vi "Calibration.vi"(8 "error in (no error)":errorcluster, 11 "Connection Data In":T2={"MX370x refnum"=refnum, "IP"="192.168.99.99", "Connection ID "=refnum, "MXCommon refnum"=refnum}) -> (0 "error out":errorcluster={"status"=TRUE, "code"=1172, "source"="Constructor Node Error creating instance of Uri in assembly System.Uri, System, Version=4.0.0.0, Culture=neutral, PublicKeyToken=b77a5c561934e089, (System.UriFormatException: Invalid URI: The hostname could not be parsed.) <append><b>System.UriFormatException</b> in MSX-E3701_dll.lvlib:Connection Open.vi->MSX-E3701_dll.lvlib:Calibration.vi"}, 3 "Connection Data Out":T2)   [LabVIEW 2014, in "MSX-E3701_dll.lvlib"]
doc: "Paanel Frontal que permite la calibracion de transductores."
uses:
  MSX-E3701_dll.lvlib
  Typedef/Connection Data.ctl
  E:/Repositorio Magnis/INF002/v0/Modules/HAL/Drivers/Sync/ADDI-DATA MSX-E3701/API/MX370x.dll
  MX370x.dll
  E:/Repositorio Magnis/INF002/v0/Modules/HAL/Drivers/Sync/ADDI-DATA MSX-E3701/API/MXCommon.dll
  MXCommon.dll
  Typedef/Calibration Data.ctl
  Typedef/Calibration Enum.ctl
panel:
  in  "Transducer Selection":u64
  in  "Desired Position":dbl format="%#_g[mm]"
  in  "Stop":bool
  out "Progress Bar":u64(slide) scale=0.0..5.0
  out "Measured value":dbl format="%#_g[mm]"
  out "Indicator":string="Leyendo los transductores de la base de datos."
  in  "Next":bool
  in  "Start":bool
  out "Cluster Calibration":T1
  # "TRANSDUCER CALIBRATION"
  # "Progress Bar"
  # "Information"
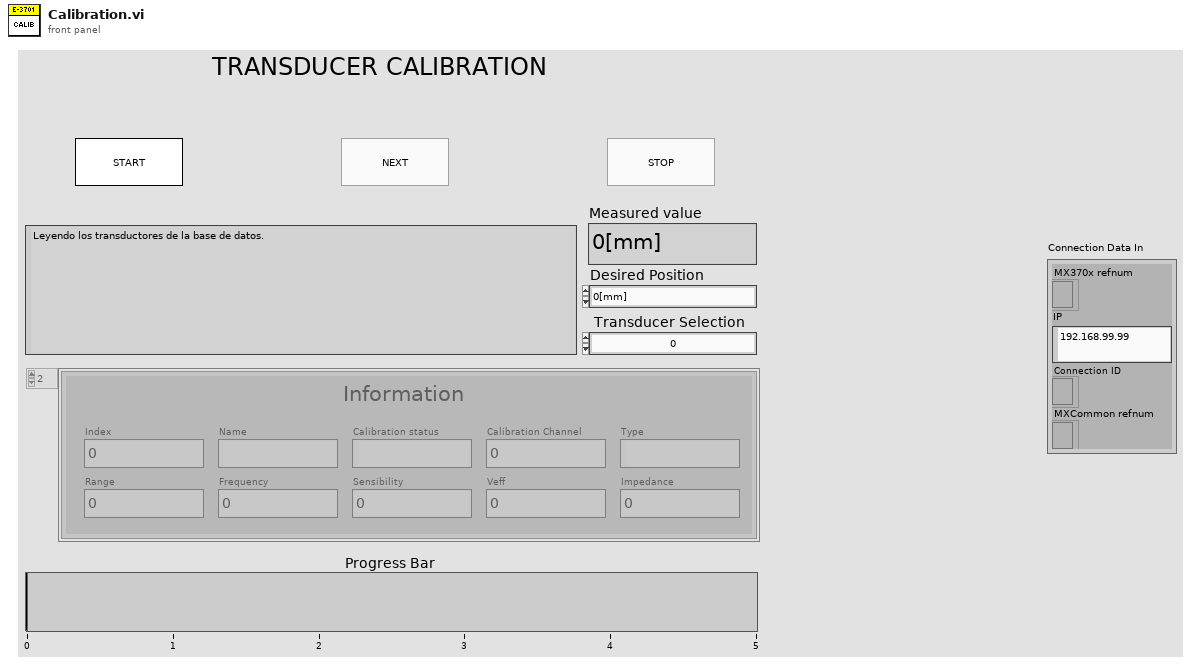
[diagram p1: front panel]
types:
  T1 = typedef "MSX-E3701_dll.lvlib/Calibration Data.ctl" = cluster{"Calibration status":string, "Name":string, "Index":u64, "Range":dbl, "Sensibility":dbl, "Veff":dbl, "Frequency":u64, "Impedance":u64, "Type":string, "Calibration Channel":u64}[]
  T2 = typedef "MSX-E3701_dll.lvlib/Connection Data.ctl" = cluster{"MX370x refnum":refnum<k24>, "IP":string, "Connection ID ":refnum<k5>, "MXCommon refnum":refnum<k24>}
  T3 = typedef "MSX-E3701_dll.lvlib/Calibration Enum.ctl" = enum16{"Init", "Idle Start", "Idle Next", "Open Web Service", "Read Transducers", "StartCalibration", "CalibrationGetCurrentStatus", "Save or Omit", "Close Web Service", "Idle Final"}
  T4 = enum8{"Enabled", "Disabled", "Disabled and Grayed Out"}
  T5 = cluster{"Calibration status":string, "Name":string, "Index":u64, "Range":dbl, "Sensibility":dbl, "Veff":dbl, "Frequency":u64, "Impedance":u64, "Type":string, "Calibration Channel":u64}
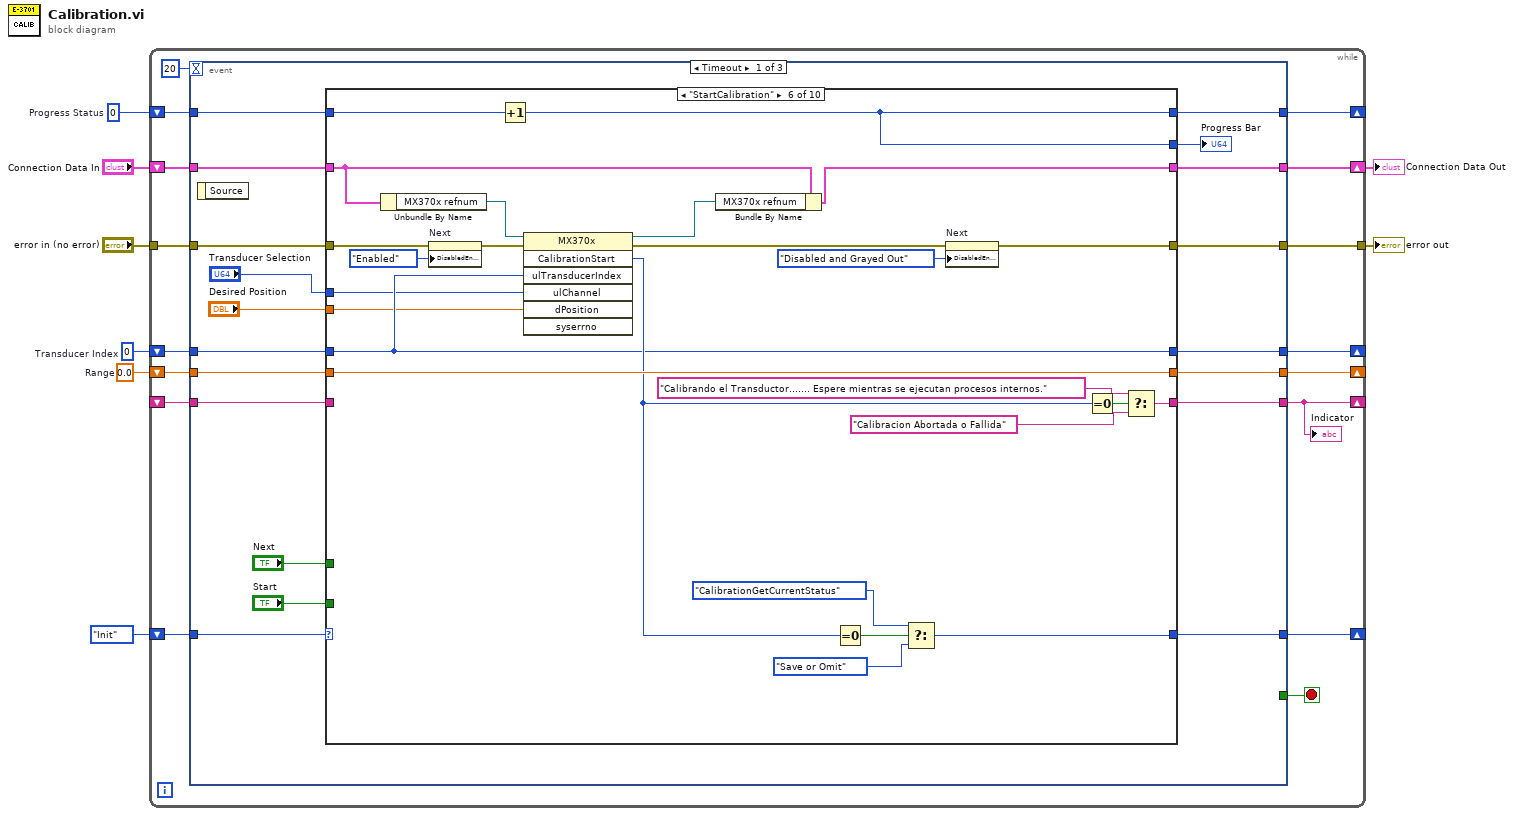
[diagram p0: block diagram]
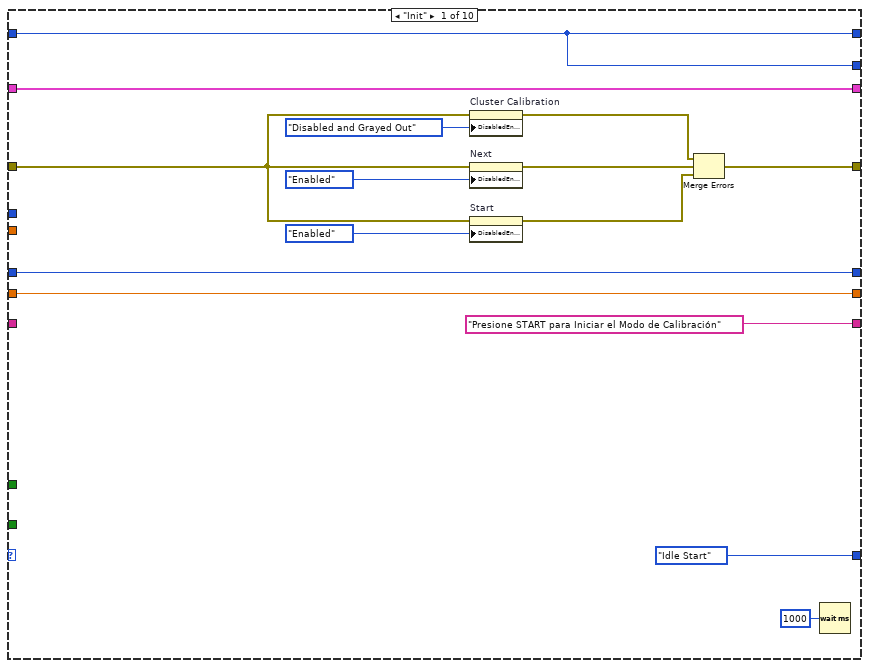
[diagram p2: hidden frame]
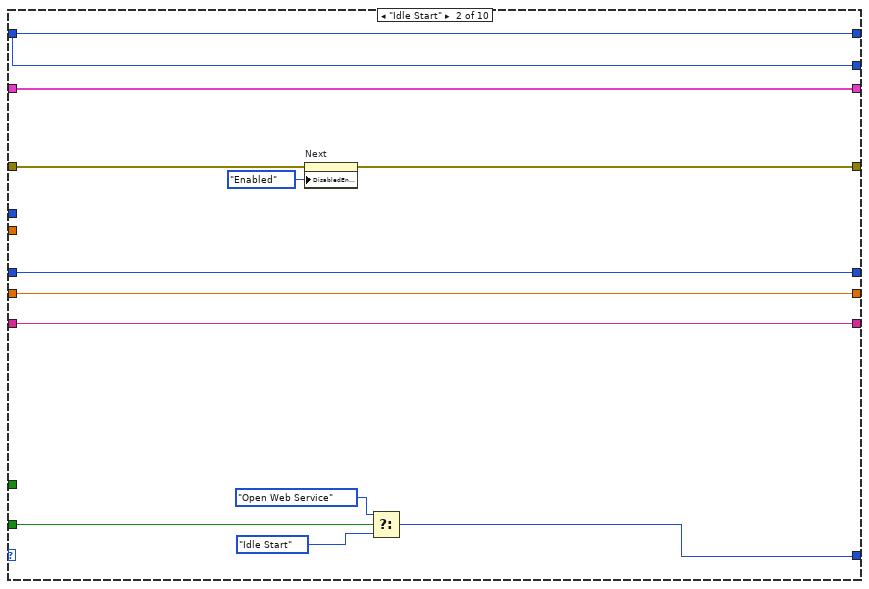
[diagram p3: hidden frame]
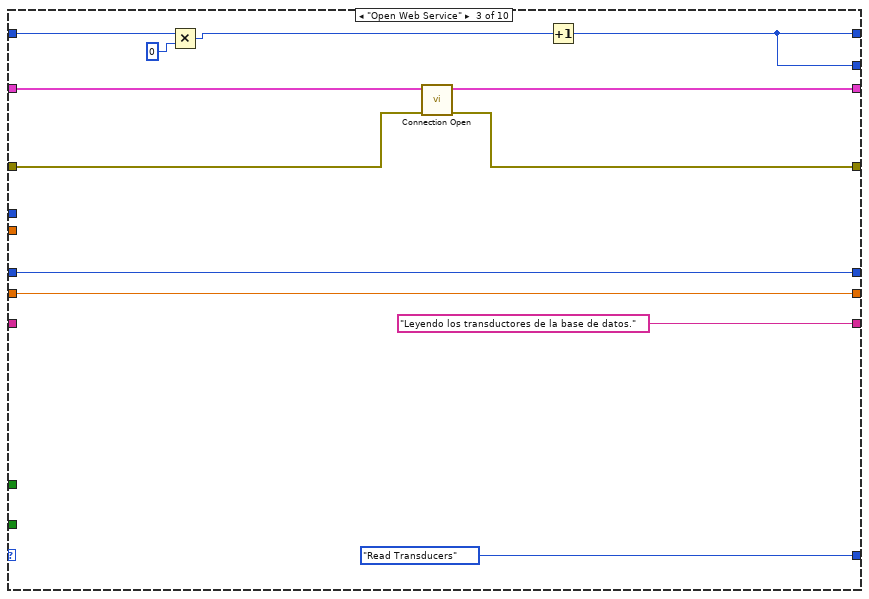
[diagram p4: hidden frame]
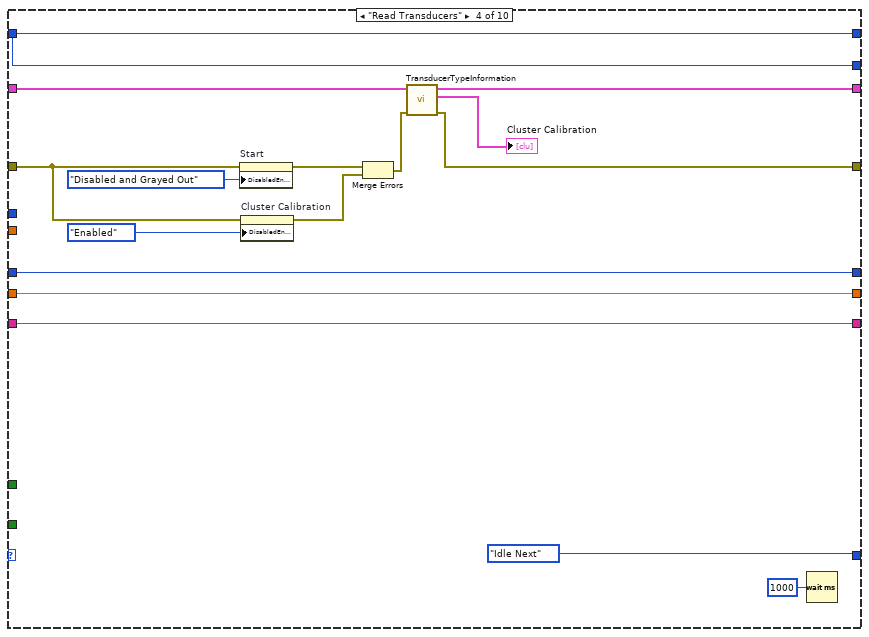
[diagram p5: hidden frame]
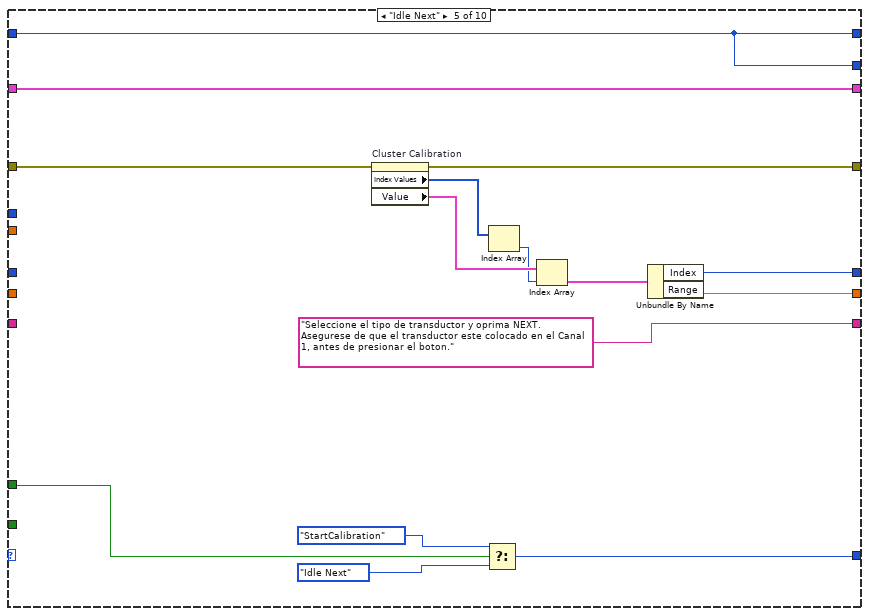
[diagram p6: hidden frame]
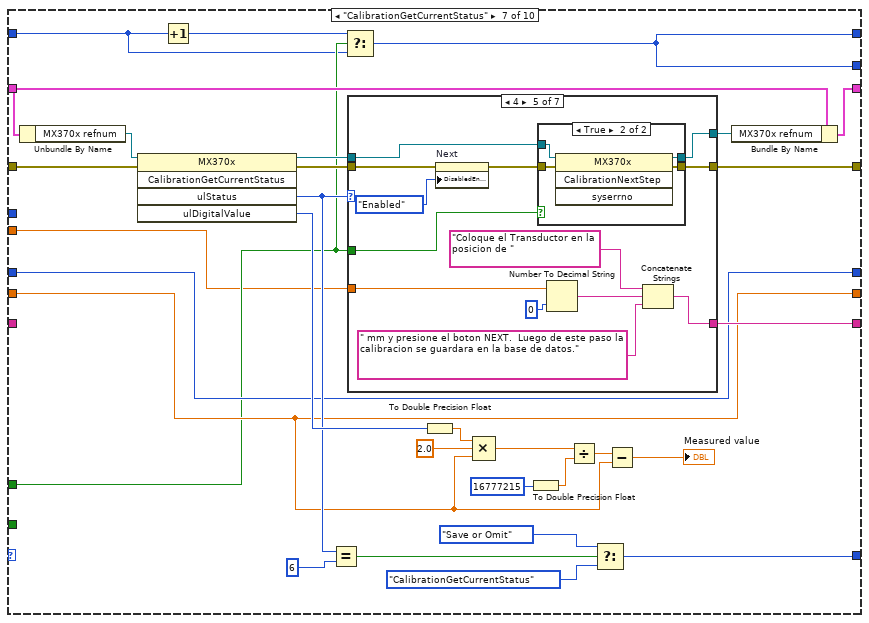
[diagram p7: hidden frame]
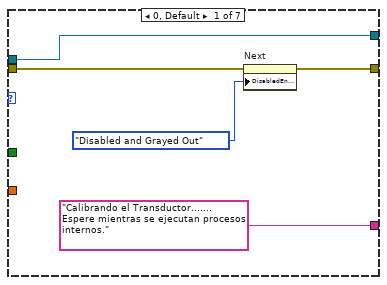
[diagram p8: hidden frame]
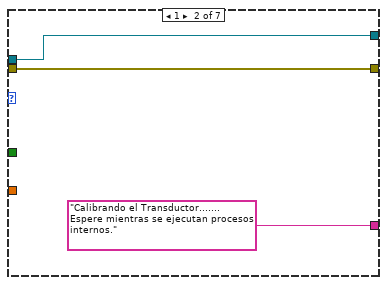
[diagram p9: hidden frame]
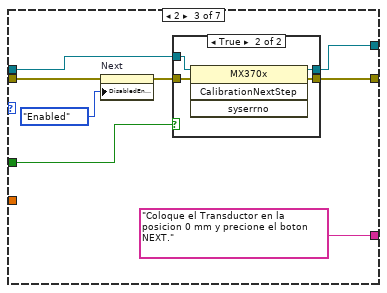
[diagram p10: hidden frame]
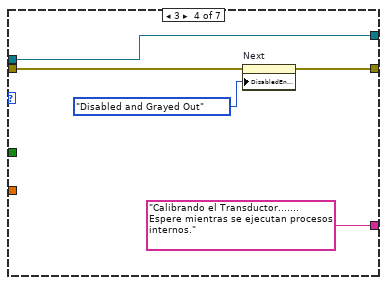
[diagram p12: hidden frame]
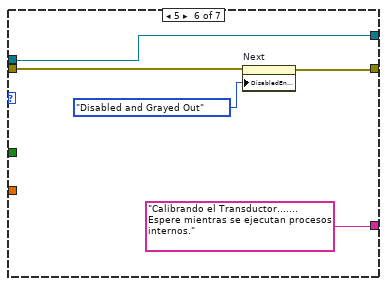
[diagram p14: hidden frame]
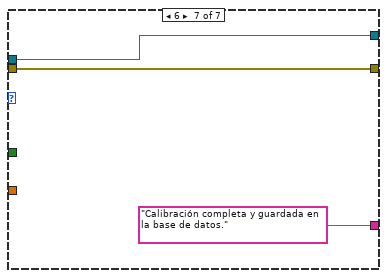
[diagram p15: hidden frame]
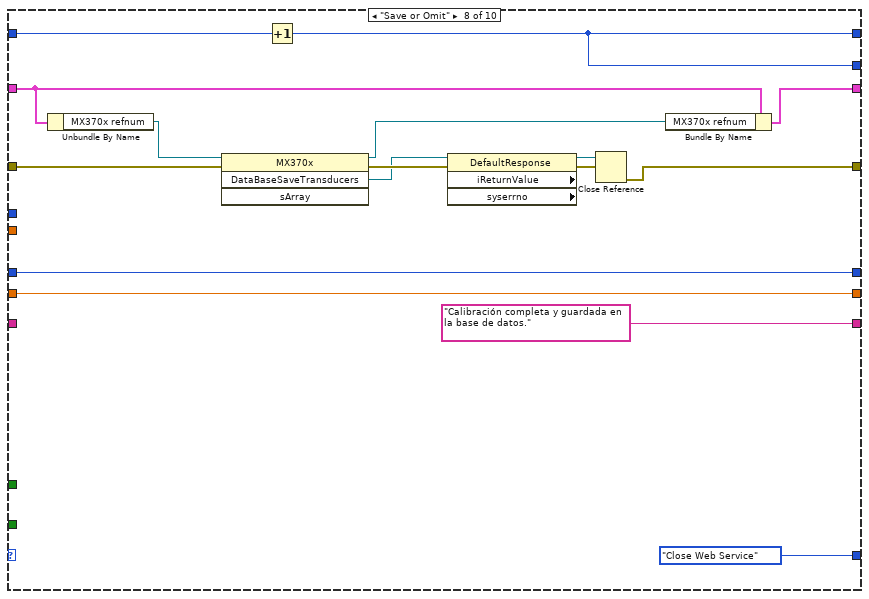
[diagram p16: hidden frame]
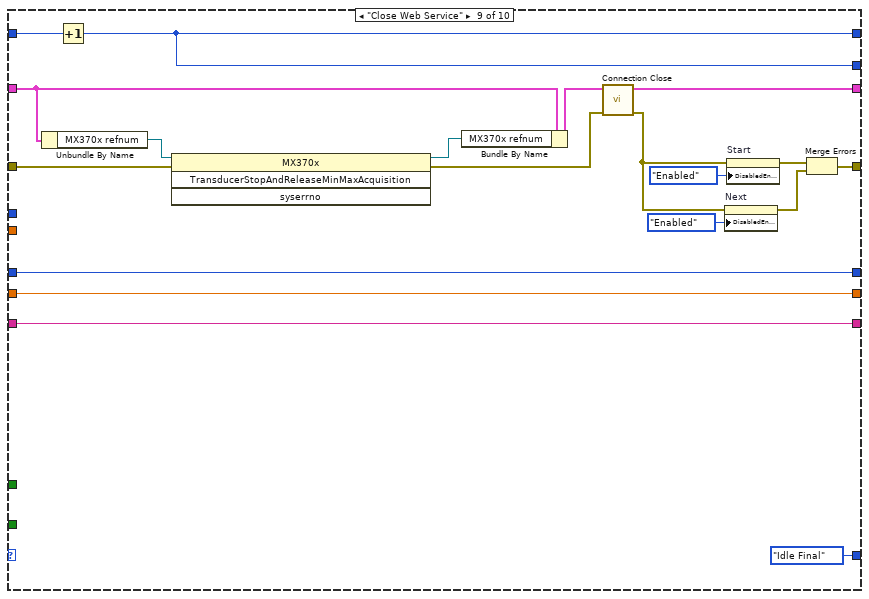
[diagram p17: hidden frame]
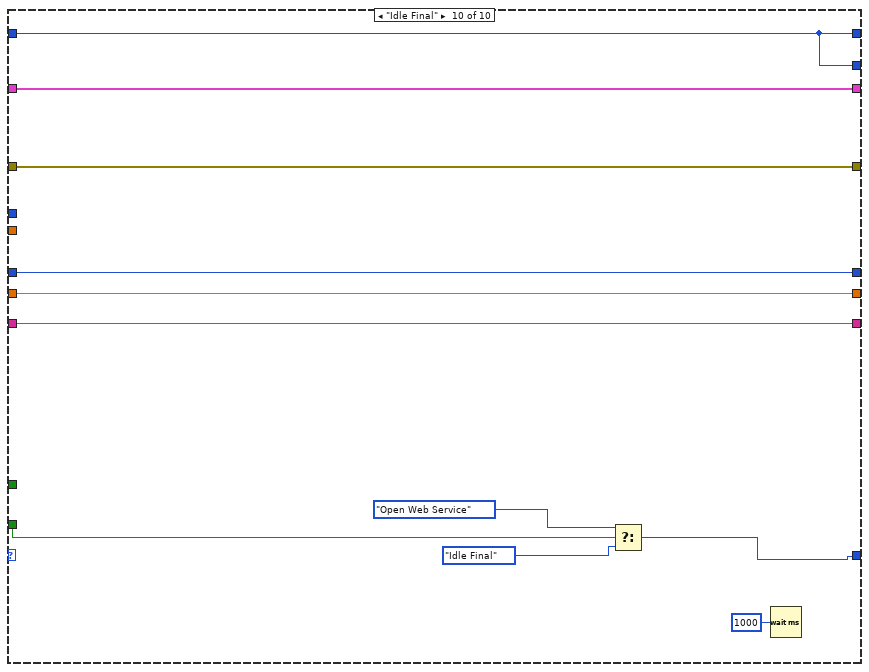
[diagram p18: hidden frame]
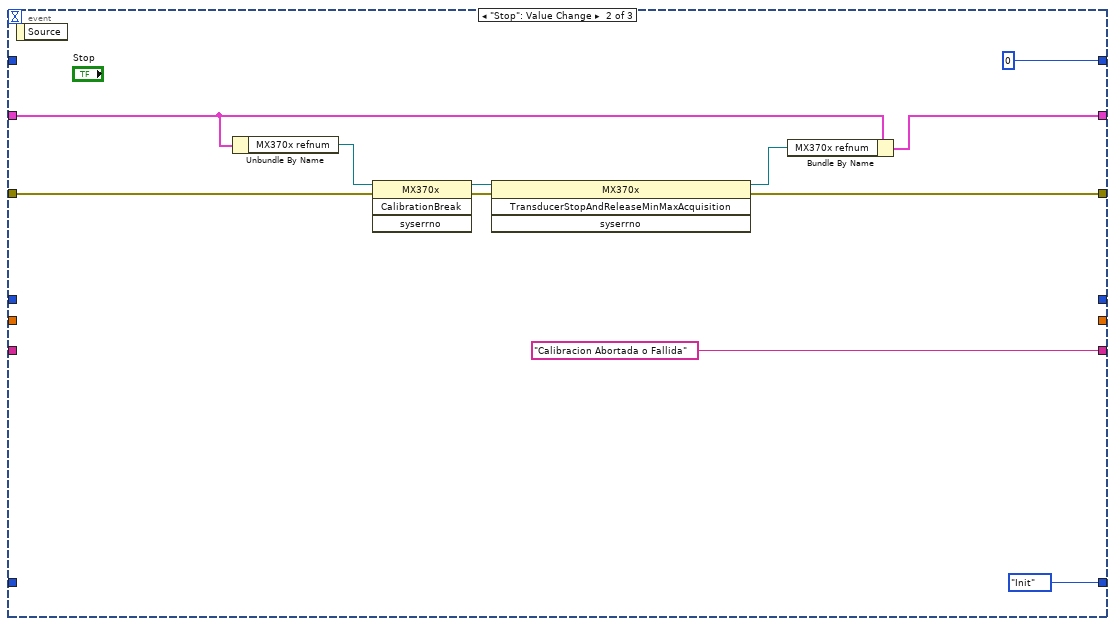
[diagram p19: hidden frame]
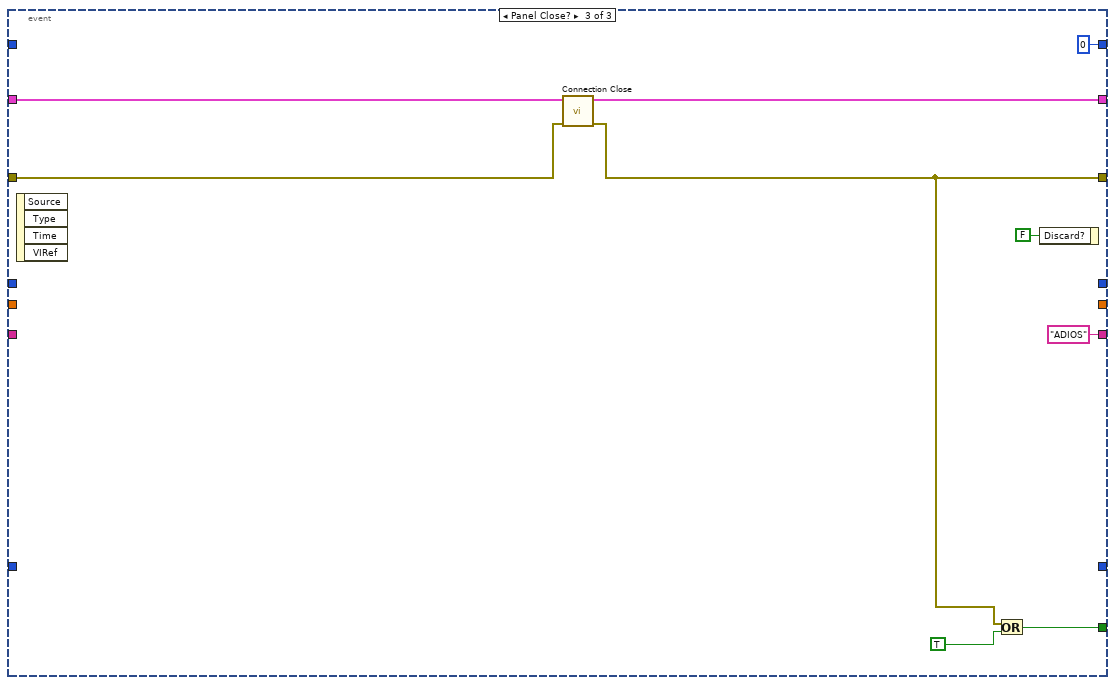
[diagram p20: hidden frame]
diagram:
  w1 = u64 0  # Progress Status
  w2 = 0.0  # Range
  w3 = u64 0  # Transducer Index
  n1 = while {
    tunnel: [w20] -> w6
    tunnel: "error in (no error)" -> [w22]
    shift-right: [w23] -> w7
    shift-left: "Connection Data In" -> [w24]
    shift-right: [w14] -> _
    shift-left: Calibration_Enum."Init" ("Enum") -> [w19]
    shift-right: [w18] -> _
    shift-left: w3 -> [w16]
    shift-right: [w17] -> _
    shift-left: w2 -> [w15]
    shift-right: [w12] -> _
    shift-left: w1 -> [w13]
    shift-right: [w10] -> _
    shift-left: _ -> [w9]
    stop <- w21 stop-if-true
    n2 = event shown="[0] Timeout" {
      selector: _ -> [_ _ _]
      dyn-events: _ -> [_ _ _]
      timeout: 20 -> [_ _ _]
      tunnel: w24 -> [w43 w278 w285]
      tunnel: [w42 w277 w284] -> w23
      tunnel: w22 -> [w41 w276 w283]
      tunnel: [_ _ w286] -> w21
      tunnel: [w40 w270 w282] -> w20
      tunnel: w19 -> [w38 _ _]
      tunnel: [w37 _ _] -> w18
      tunnel: [w36 _ _] -> w17
      tunnel: w16 -> [w35 _ _]
      tunnel: w15 -> [w34 _ _]
      tunnel: [w33 Calibration_Enum."Init" ("Enum") _] -> w14
      tunnel: w13 -> [w31 _ _]
      tunnel: [w30 u64 0 ("Progress Status") u64 0 ("Progress Status")] -> w12
      tunnel: [w28 "Calibracion Abortada o Fallida" ("Caption.Text") "ADIOS" ("Caption.Text")] -> w10
      tunnel: w9 -> [w27 _ _]
      event Timeout {
        n3 = event-data() -> ()  [unwired: 1 in, 1 out]
        n4 = case shown="\"StartCalibration\"" w38 {
          tunnel: w43 -> [w54 w70 w82 w98 w110 w137 w168 w236 w243 w268]
          tunnel: [w54 w70 w81 w97 w110 w135 w167 w235 w257 w268] -> w42
          tunnel: [w55 w61 w80 w96 w109 w117 w149 w234 w247 w267] -> w40
          tunnel: w41 -> [w50 w62 w79 w89 w100 w132 w166 w233 w245 w267]
          tunnel: [Calibration_Enum."Idle Start" ("Enum") w60 Calibration_Enum."Read Transducers" ("f") Calibration_Enum."Idle Next" ("Enum") w99 w116 w140 Calibration_Enum."Close Web Service" ("Enum") Calibration_Enum."Idle Final" ("Enum") w261] -> w33
          tunnel: "Start" -> [_ w68 _ _ _ _ _ _ _ w263]
          tunnel: [w48 w66 w78 w88 w102 w122 w145 w227 w255 w266] -> w37
          tunnel: [w47 w65 w77 w87 w107 w131 w146 w231 w254 w265] -> w36
          tunnel: w35 -> [w48 w66 w78 w88 _ w122 w145 w227 w255 w266]
          tunnel: w34 -> [w47 w65 w77 w87 _ w131 w146 w231 w254 w265]
          tunnel: ["Presione START para Iniciar el Modo de Calibración" ("Indicator") w59 "Leyendo los transductores de la base de datos." ("Indicator") w83 "Seleccione el tipo de transductor y oprima NEXT. Asegurese de que el transductor este colocado en el Canal 1, antes de presionar el boton." ("Caption.Text") w124 w147 "Calibración completa y guardada en la base de datos." ("Caption.Text") w239 w259] -> w28
          tunnel: "Next" -> [_ _ _ _ w103 _ w143 _ _ _]
          tunnel: [w46 w64 w75 w85 w101 w120 w144 w228 w240 w260] -> w30
          tunnel: w31 -> [w46 w64 w73 w85 w101 w121 w141 w229 w252 w260]
          tunnel: [w46 w64 w75 w85 w101 w120 w144 w228 w240 w260] -> w29
          tunnel: w27 -> [_ w59 _ w83 _ _ _ _ w239 w259]
          tunnel: "Desired Position" -> [_ _ _ _ _ w115 w139 _ _ _]
          tunnel: "Transducer Selection" -> [_ _ _ _ _ w114 _ _ _ _]
          frame "Init" {
            n5 = property on="Cluster Calibration" class="Arr (strict)"(error in=w50, "DisabledEnum"=T4."Disabled and Grayed Out" ("Disabled")) -> (error out=w56:errorcluster)  [unwired: 1 in, 1 out]
            n6 = property on="Next" class="Bool"(error in=w50, "DisabledEnum"=T4."Enabled" ("Disabled")) -> (error out=w52:errorcluster)  [unwired: 1 in, 1 out]
            n7 = property on="Start" class="Bool"(error in=w50, "DisabledEnum"=T4."Enabled" ("Disabled")) -> (error out=w51:errorcluster)  [unwired: 1 in, 1 out]
            n8 = Merge Errors(w56, w52, w51) -> (w55:errorcluster)
            n9 = Wait (ms)(milliseconds to wait=u32 1000) -> ()  [unwired: 1 out]
          }
          frame "Idle Start" {
            n10 = property on="Next" class="Bool"(error in=w62, "DisabledEnum"=T4."Enabled" ("Disabled")) -> (error out=w61:errorcluster)  [unwired: 1 in, 1 out]
            n11 = Select(t=Calibration_Enum."Open Web Service" ("Enum"), s=w68, f=Calibration_Enum."Idle Start") -> (s? t:f=w60:T3)
          }
          frame "Open Web Service" {
            n12 = Multiply(x=w73, y=u64 0) -> (x*y=w74:u64)
            n13 = call "Connection Open.vi"("Error In"=w79, "Connection Data In"=w82) -> ("Error Out"=w80:errorcluster, "Connection Data Out"=w81:T2)  [unwired: 8 in]
            n14 = Increment(x=w74) -> (x+1=w75:u64)
          }
          frame "Read Transducers" {
            n15 = property on="Start" class="Bool"(error in=w89, "DisabledEnum"=T4."Disabled and Grayed Out" ("Disabled")) -> (error out=w92:errorcluster)  [unwired: 1 in, 1 out]
            n16 = property on="Cluster Calibration" class="Arr (strict)"(error in=w89, "DisabledEnum"=T4."Enabled" ("Disabled")) -> (error out=w91:errorcluster)  [unwired: 1 in, 1 out]
            n17 = Merge Errors(w92, w91) -> (w90:errorcluster)
            n18 = call "TransducerTypeInformation.vi"("error in (no error)"=w90, "Connection Data In"=w98) -> ("error out"=w96:errorcluster, "Cluster Calibration"=→"Cluster Calibration":T1, "Connection Data Out"=w97:T2)  [unwired: 7 in]
            n19 = Wait (ms)(milliseconds to wait=u32 1000) -> ()  [unwired: 1 out]
          }
          frame "Idle Next" {
            n20 = property on="Cluster Calibration" class="Arr (strict)"(error in=w100) -> (error out=w109:errorcluster, "Index Values"=w113:u32[], "Value"=w112:T1)  [unwired: 1 in, 1 out]
            n21 = Select(t=Calibration_Enum."StartCalibration" ("Enum"), s=w103, f=Calibration_Enum."Idle Next") -> (s? t:f=w99:T3)
            n22 = Index Array(array=w113) -> (element=w108:u32)  [unwired: 1 in]
            n23 = Index Array(array=w112, index=w108) -> (element=w111:T5)
            n24 = Unbundle By Name(w111) -> ("Index"=w102:u64, "Range"=w107:dbl)
          }
          frame "StartCalibration" {
            n25 = Unbundle By Name(w137) -> ("MX370x refnum"=w138:refnum<k24>)
            n26 = property on="Next" class="Bool"(error in=w132, "DisabledEnum"=T4."Enabled" ("Disabled")) -> (error out=w133:errorcluster)  [unwired: 1 in, 1 out]
            n27 = Increment(x=w121) -> (x+1=w120:u64)
            n28 = invoke class="MX370x" method="CalibrationStart"(reference=w138, error in=w133, "ulTransducerIndex"=w122, "ulChannel"=w114, "dPosition"=w115) -> (reference out=w136:refnum<k24>, error out=w118:errorcluster, "CalibrationStart"=w126:i32)  [unwired: 2 in, 4 out]
            n29 = Bundle By Name(cluster=w137, "MX370x refnum"=w136) -> (w135:T2)
            n30 = Equal To 0?(x=w126) -> (x = 0?=w130:bool)
            n31 = Select(t=Calibration_Enum."CalibrationGetCurrentStatus" ("Enum"), s=w130, f=Calibration_Enum."Save or Omit" ("Enum")) -> (s? t:f=w116:T3)
            n32 = property on="Next" class="Bool"(error in=w118, "DisabledEnum"=T4."Disabled and Grayed Out" ("Disabled")) -> (error out=w117:errorcluster)  [unwired: 1 in, 1 out]
            n33 = Equal To 0?(x=w126) -> (x = 0?=w127:bool)
            n34 = Select(t="Calibrando el Transductor....... Espere mientras se ejecutan procesos internos." ("Caption.Text"), s=w127, f="Calibracion Abortada o Fallida") -> (s? t:f=w124:string)
          }
          frame "CalibrationGetCurrentStatus" {
            n35 = Unbundle By Name(w168) -> ("MX370x refnum"=w165:refnum<k24>)
            n36 = invoke class="MX370x" method="CalibrationGetCurrentStatus"(reference=w165, error in=w166) -> (reference out=w150:refnum<k24>, error out=w151:errorcluster, "ulStatus"=w156:u64, "ulDigitalValue"=w160:u64)  [unwired: 3 in, 1 out]
            n37 = Increment(x=w141) -> (x+1=w142:u64)
            n38 = Equal?(x=w156, y=u64 6) -> (x = y?=w154:bool)
            n39 = Select(t=w142, s=w143, f=w141) -> (s? t:f=w144:u64)
            n40 = case shown="4" w156 {
              tunnel: w151 -> [w172 w176 w179 w194 w204 w218 w220]
              tunnel: w150 -> [w170 w175 w180 w191 w205 w216 w222]
              tunnel: [w171 w176 w184 w193 w203 w217 w220] -> w149
              tunnel: [w170 w175 w183 w191 w197 w216 w222] -> w148
              tunnel: ["Calibrando el Transductor....... Espere mientras se ejecutan procesos internos." ("Caption.Text") "Calibrando el Transductor....... Espere mientras se ejecutan procesos internos." ("Caption.Text") "Coloque el Transductor en la posicion 0 mm y precione el boton NEXT." ("Caption.Text") "Calibrando el Transductor....... Espere mientras se ejecutan procesos internos." ("Caption.Text") w198 "Calibrando el Transductor....... Espere mientras se ejecutan procesos internos." ("Caption.Text") "Calibración completa y guardada en la base de datos." ("Caption.Text")] -> w147
              tunnel: w143 -> [_ _ w177 _ w206 _ _]
              tunnel: w139 -> [_ _ _ _ w196 _ _]
              frame 0, Default {
                n41 = property on="Next" class="Bool"(error in=w172, "DisabledEnum"=T4."Disabled and Grayed Out" ("Disabled")) -> (error out=w171:errorcluster)  [unwired: 1 in, 1 out]
              }
              frame 1 {
              }
              frame 2 {
                n42 = property on="Next" class="Bool"(error in=w179, "DisabledEnum"=T4."Enabled" ("Disabled")) -> (error out=w181:errorcluster)  [unwired: 1 in, 1 out]
                n43 = case shown="True" w177 {
                  tunnel: [w185 w190] -> w184
                  tunnel: [w186 w189] -> w183
                  tunnel: w181 -> [w185 w188]
                  tunnel: w180 -> [w186 w187]
                  frame False {
                  }
                  frame True {
                    n44 = invoke class="MX370x" method="CalibrationNextStep"(reference=w187, error in=w188) -> (reference out=w189:refnum<k24>, error out=w190:errorcluster)  [unwired: 2 in, 2 out]
                  }
                }
              }
              frame 3 {
                n45 = property on="Next" class="Bool"(error in=w194, "DisabledEnum"=T4."Disabled and Grayed Out" ("Disabled")) -> (error out=w193:errorcluster)  [unwired: 1 in, 1 out]
              }
              frame 4 {
                n46 = property on="Next" class="Bool"(error in=w204, "DisabledEnum"=T4."Enabled" ("Disabled")) -> (error out=w208:errorcluster)  [unwired: 1 in, 1 out]
                n47 = case shown="True" w206 {
                  tunnel: [w209 w214] -> w203
                  tunnel: [w210 w213] -> w197
                  tunnel: w208 -> [w209 w212]
                  tunnel: w205 -> [w210 w211]
                  frame False {
                  }
                  frame True {
                    n48 = invoke class="MX370x" method="CalibrationNextStep"(reference=w211, error in=w212) -> (reference out=w213:refnum<k24>, error out=w214:errorcluster)  [unwired: 2 in, 2 out]
                  }
                }
                n49 = Number To Decimal String(number=w196, width (-)=i16 0) -> (decimal integer string=w201:string)
                n50 = Concatenate Strings("Coloque el Transductor en la posicion de " ("Caption.Text"), w201, " mm y presione el boton NEXT.  Luego de este paso la calibracion se guardara en la base de datos.") -> (w198:string)
              }
              frame 5 {
                n51 = property on="Next" class="Bool"(error in=w218, "DisabledEnum"=T4."Disabled and Grayed Out" ("Disabled")) -> (error out=w217:errorcluster)  [unwired: 1 in, 1 out]
              }
              frame 6 {
              }
            }
            n52 = To Double Precision Float(number=w160) -> (double precision float=w159:dbl)
            n53 = Compound Arithmetic op=MULTIPLY(w159, 2.0 ("x"), w146) -> (w161:dbl)
            n54 = To Double Precision Float(number=u64 16777215 ("x")) -> (double precision float=w157:dbl)
            n55 = Divide(x=w161, y=w157) -> (x/y=w162:dbl)
            n56 = Select(t=Calibration_Enum."Save or Omit" ("Enum"), s=w154, f=Calibration_Enum."CalibrationGetCurrentStatus" ("Enum")) -> (s? t:f=w140:T3)
            n57 = Subtract(x=w162, y=w146) -> (x-y=→"Measured value":dbl)
            n58 = Bundle By Name(cluster=w168, "MX370x refnum"=w148) -> (w167:T2)
          }
          frame "Save or Omit" {
            n59 = Unbundle By Name(w236) -> ("MX370x refnum"=w238:refnum<k24>)
            n60 = invoke class="MX370x" method="DataBaseSaveTransducers"(reference=w238, error in=w233) -> (reference out=w237:refnum<k24>, error out=w224:errorcluster, "DataBaseSaveTransducers"=w223:refnum<k24>)  [unwired: 2 in, 1 out]
            n61 = Increment(x=w229) -> (x+1=w228:u64)
            n62 = property class="DefaultResponse" props=["iReturnValue", "syserrno"](reference=w223, error in=w224) -> (reference out=w225:refnum<k24>, error out=w226:errorcluster)  [unwired: 2 out]
            n63 = Close Reference(reference=w225, error in (no error)=w226) -> (error out=w234:errorcluster)
            n64 = Bundle By Name(cluster=w236, "MX370x refnum"=w237) -> (w235:T2)
          }
          frame "Close Web Service" {
            n65 = Unbundle By Name(w243) -> ("MX370x refnum"=w246:refnum<k24>)
            n66 = Increment(x=w252) -> (x+1=w240:u64)
            n67 = invoke class="MX370x" method="TransducerStopAndReleaseMinMaxAcquisition"(reference=w246, error in=w245) -> (reference out=w241:refnum<k24>, error out=w244:errorcluster)  [unwired: 2 in, 2 out]
            n68 = Bundle By Name(cluster=w243, "MX370x refnum"=w241) -> (w242:T2)
            n69 = call "Connection Close.vi"("error in (no error)"=w244, "Connection Data In"=w242) -> ("error out"=w250:errorcluster, "Connection Data Out"=w257:T2)  [unwired: 8 in]
            n70 = property on="Next" class="Bool"(error in=w250, "DisabledEnum"=T4."Enabled" ("Disabled")) -> (error out=w249:errorcluster)  [unwired: 1 in, 1 out]
            n71 = property on="Start" class="Bool"(error in=w250, "DisabledEnum"=T4."Enabled" ("Disabled")) -> (error out=w248:errorcluster)  [unwired: 1 in, 1 out]
            n72 = Merge Errors(w248, w249) -> (w247:errorcluster)
          }
          frame "Idle Final" {
            n73 = Select(t=Calibration_Enum."Open Web Service", s=w263, f=Calibration_Enum."Idle Final" ("Enum")) -> (s? t:f=w261:T3)
            n74 = Wait (ms)(milliseconds to wait=u32 1000) -> ()  [unwired: 1 out]
          }
        }
        "Progress Bar" <- w29
      }
      event "Stop": Value Change {
        n75 = event-data() -> ()  [unwired: 1 in, 1 out]
        n76 = Unbundle By Name(w278) -> ("MX370x refnum"=w279:refnum<k24>)
        n77 = invoke class="MX370x" method="CalibrationBreak"(reference=w279, error in=w276) -> (reference out=w272:refnum<k24>, error out=w271:errorcluster)  [unwired: 2 in, 2 out]
        n78 = invoke class="MX370x" method="TransducerStopAndReleaseMinMaxAcquisition"(reference=w272, error in=w271) -> (reference out=w269:refnum<k24>, error out=w270:errorcluster)  [unwired: 2 in, 2 out]
        n79 = Bundle By Name(cluster=w278, "MX370x refnum"=w269) -> (w277:T2)
      }
      event Panel Close? {
        n80 = event-data() -> ()  [unwired: 1 in, 4 out]
        n81 = call "Connection Close.vi"("error in (no error)"=w283, "Connection Data In"=w285) -> ("error out"=w282:errorcluster, "Connection Data Out"=w284:T2)  [unwired: 8 in]
        n82 = Or(x=w282, y=TRUE) -> (x .or. y?=w286:bool)
        n83 = event-data("Discard?"=FALSE) -> ()  [unwired: 1 in, 1 out]
      }
    }
    "Indicator" <- w10
  }
  "error out" <- w6
  "Connection Data Out" <- w7
